vi "Qcorrect.vi"(2 "Subtract Q curve":bool, 3 "Nstep":i16, 4 "Max Gain":bool, 5 "Amp of Q curve":dbl, 6 "Step Width (MHz)":dbl, 7 "Center Freq (MHz)":dbl) -> (0 "Start":i32, 1 "Array":dbl[](array[numeric]))   [LabVIEW 2018]
panel:
  # "Calculates Q curve correction and\npedestal slope correction"
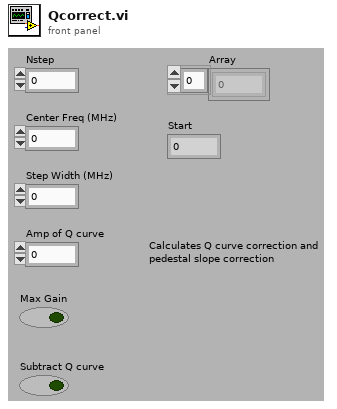
[diagram p1: front panel]
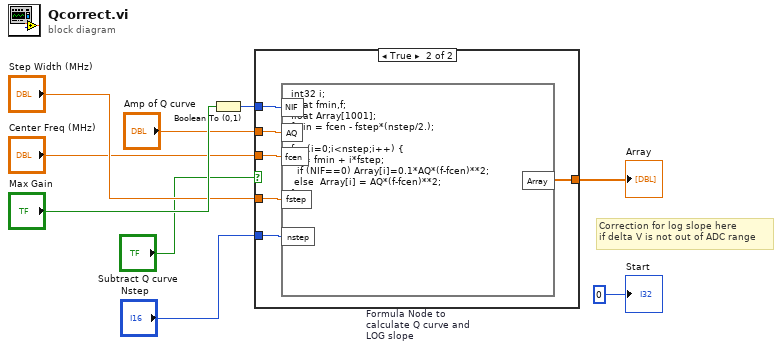
[diagram p0: block diagram]
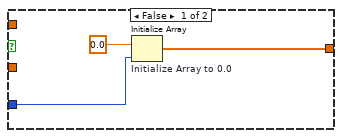
[diagram p2: hidden frame]
diagram:
  # "Correction for log slope here\nif delta V is not out of ADC range"
  n1 = Boolean To (0,1)(Boolean="Max Gain") -> (0, 1=w3:i16)
  n2 = case shown="True" "Subtract Q curve" {
    tunnel: [w10 w18] -> w1
    tunnel: "Center Freq (MHz)" -> [_ w17]
    tunnel: w3 -> [_ w16]
    tunnel: "Step Width (MHz)" -> [_ w15]
    tunnel: "Nstep" -> [w12 w14]
    tunnel: "Amp of Q curve" -> [_ w13]
    frame False {
      n3 = Initialize Array "Initialize Array to 0.0"(0.0, w12) -> (w10:dbl[])
    }
    frame True {
      n4 = formula code="int32 i;\nfloat fmin,f;\nfloat Array[1001];\nfmin = fcen - fstep*(nstep/2.);\n\nfor (i=0;i<nstep;i++) {\n  f = fmin + i*fstep;\n  if (NIF==0) Array[i]=0.1*AQ*(f-fcen)**2;\n else  Array[i] = AQ*(f-fcen)**2;\n}" "Formula Node to calculate Q curve and LOG slope"("fcen"=w17, "fstep"=w15, "nstep"=w14, "NIF"=w16, "AQ"=w13) -> ("Array"=w18:dbl[])
    }
  }
  "Array" <- w1
  "Start" <- 0
